vi "MALT160T Output Get Several.vi"(8 "error in":errorcluster, 9 "Port":i32, 10 "Address":i32, 11 "MALT CardType":T1=enum."MALT132") -> (3 "Status":u8[](array[numeric]) format="%02x")   [LabVIEW 2018, in "AltonTech MALT200817.lvlib"]
uses:
  <instrlib>/AltonTech MALT/AltonTech MALT200817.lvlib
  <instrlib>/AltonTech MALT/Public/Types/MALT CardTypes.ctl
panel:
  out "error out":errorcluster
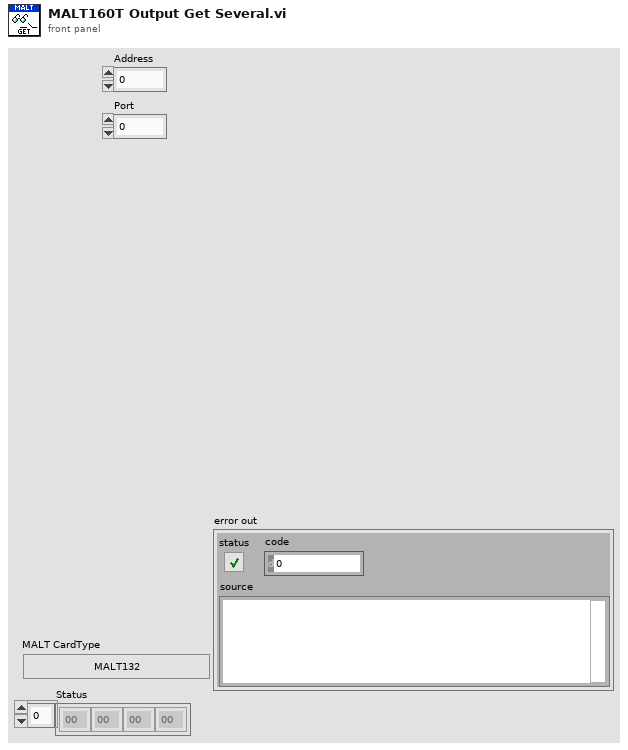
[diagram p1: front panel]
types:
  T1 = typedef "AltonTech MALT200817.lvlib/MALT CardTypes.ctl" = enum32{"-", "YAV90832", "YAV904X8", "MALT132", "YAV91616", "YAV90PIN", "YAV90096", "YAV90HVT", "YAV90CLR", "YAV90128", "YAV90PNE", "YAVCANCON", "YAV91775", "YAV90XXX", "YAV90MMU", "H730050", "H710060", "H710061", "YAV90304", "MMI", "YAV90060", "MALT160T", "YAV90059", "Not Defined"}
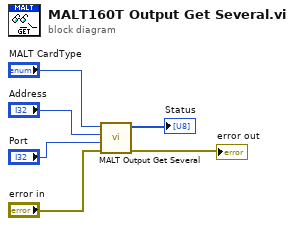
[diagram p0: block diagram]
diagram:
  n1 = call <instrlib>:"MALT Output Get Several.vi"("error in"="error in", "Port"="Port", "Address"="Address", "MALT CardType"="MALT CardType") -> ("error out"=→"error out":errorcluster, "Status Map"=→"Status":u8[])  [unwired: 6 in]
